vi "Set Virtual Axis Speed (Polymorphic).vi"   [LabVIEW 2018, in "Zaber A Series.lvlib"]
doc: "Sets the maximum speed of a virtual axis that was previously created using the Create Virtual Axis VI. The speed is specified in native device speed units - use the Convert Velocity Units to Device Units VI to convert from standard units.\n\nThis VI requires that the Initialize VI has been called with the same serial port and that the specified virtual axis exists."
uses:
  Zaber A Series.lvlib
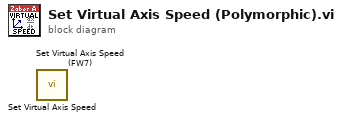
[diagram p0: block diagram]
diagram:
  n1 = call "Set Virtual Axis Speed.vi"() -> ()  [unwired: 10 in, 2 out]
  n2 = call "Set Virtual Axis Speed (FW7).vi"() -> ()  [unwired: 10 in, 2 out]
